vi "shared_Create Error.vi"(8 "error in (no error)":errorcluster, 11 "error code (0)":i32) -> (0 "error out":errorcluster)   [LabVIEW 2011]
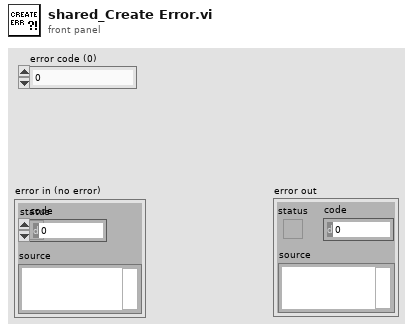
[diagram p1: front panel]
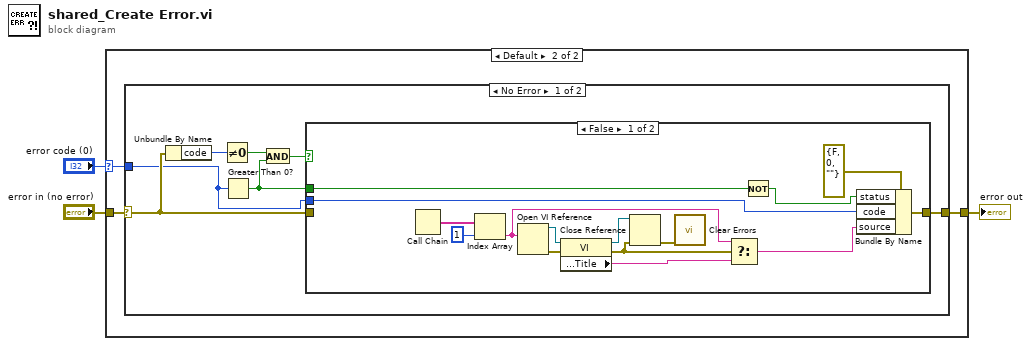
[diagram p0: block diagram]
diagram:
  n1 = case shown="Default" "error code (0)" {
    selector: "error code (0)" -> [_ w5]
    tunnel: [w4 w7] -> w3
    tunnel: "error in (no error)" -> [w4 w6]
    frame 0 {
      # "If the error code in equals zero, then propagate the error in cluster regardless of its value."
    }
    frame Default {
      n2 = case shown="No Error" w6 {
        selector: w6 -> [w11 w31]
        tunnel: [w14 w31] -> w7
        tunnel: w5 -> [w10 _]
        frame No Error {
          n3 = Unbundle By Name(w11) -> ("code"=w13:i32)
          n4 = Not Equal To 0?(x=w13) -> (x != 0?=w9:bool)
          n5 = Greater Than 0?(x=w10) -> (x > 0?=w8:bool)
          n6 = And(x=w9, y=w8) -> (x .and. y?=w12:bool)
          n7 = case shown="False" w12 {
            tunnel: [w29 w30] -> w14
            tunnel: w10 -> [w26 _]
            tunnel: w11 -> [_ w30]
            tunnel: w8 -> [w17 _]
            frame False {
              n8 = Call Chain() -> (call chain=w21:string[])
              n9 = Index Array(array=w21, index=1) -> (element=w19:string)
              n10 = Open VI Reference(vi path=w19) -> (vi reference=w24:refnum<vi>, error out=w23:errorcluster)  [unwired: 5 in]
              n11 = property class="VI"(reference=w24, error in=w23) -> (reference out=w22:refnum<vi>, error out=w20:errorcluster, "Front Panel Window:Title"=w18:string)
              n12 = Close Reference(reference=w22, error in (no error)=w20) -> (error out=w15:errorcluster)
              n13 = call <vilib>:"Clear Errors.vi"("error in (no error)"=w15) -> ()  [unwired: 6 in, 1 out]
              n14 = Select(t=w19, s=w20, f=w18) -> (s? t:f=w16:string)
              n15 = Not(x=w17) -> (.not. x?=w27:bool)
              n16 = Bundle By Name(cluster=errorcluster {"status"=FALSE, "code"=0, "source"=""} ("error out"), "status"=w27, "code"=w26, "source"=w16) -> (w29:errorcluster)
            }
            frame True {
              # "If the error code input is setting a warning, and a warning is already set on the wire, then we\ngo with the one already on the wire."
            }
          }
        }
        frame Error {
          # "An error in trumps any error code input."
        }
      }
    }
  }
  "error out" <- w3
